vi "Temperature User Interface.vi"() -> ()   [LabVIEW 2023, in "GUI.lvlib" / "Diagnostic.lvlib"]
uses:
  Diagnostic.lvlib
  HardwareAbstractionLayer_LVOOP/Modbus/Modbus_class/Modbus.lvclass
  HardwareAbstractionLayer_LVOOP/Database/SQL Public VI/Control/DB Options.ctl
  HardwareAbstractionLayer_LVOOP/Main/Class Ref.ctl
  HardwareAbstractionLayer_LVOOP/DMM/DMM.lvclass
  HardwareAbstractionLayer_LVOOP/Function Generator/Function Generator.lvclass
  HardwareAbstractionLayer_LVOOP/Oscilloscope/Oscilloscope.lvclass
  HardwareAbstractionLayer_LVOOP/PowerSupply/PowerSupply.lvclass
  HardwareAbstractionLayer_LVOOP/Teststand/Teststand.lvclass
  HardwareAbstractionLayer_LVOOP/Analog Output/AO/AO.lvclass
  HardwareAbstractionLayer_LVOOP/Analog Input/AI/AI.lvclass
  HardwareAbstractionLayer_LVOOP/Database/Database.lvclass
  HardwareAbstractionLayer_LVOOP/Digital Output/DO_class/DO.lvclass
  HardwareAbstractionLayer_LVOOP/Digital Input/DI_class/DI.lvclass
  HardwareAbstractionLayer_LVOOP/PWM Output/PWM Output_class/PWM Output.lvclass
  HardwareAbstractionLayer_LVOOP/PWM Input/PWM Input_class/PWM Input.lvclass
  HardwareAbstractionLayer_LVOOP/NI Switch/NISwitch_class/NISwitch.lvclass
  HardwareAbstractionLayer_LVOOP/CAN/CAN Lib/CAN_class/CAN.lvclass
  HardwareAbstractionLayer_LVOOP/Main/Main.lvclass
panel:
  out "Holding Registers Value":u16[](array[numeric])
  in  "Slave unit ID":u8=1
  out "error out":errorcluster
  in  "Modbus RTU":T1={"unit ID"=1, "serial type"=enum."RTU", "baud rate"=9600, "parity (even)"=2, "flow control (none)"=0, "VISA resource name"=""} {"flow control (none)" items=["None", "XON/XOFF", "RTS/CTS", "XON/XOFF & RTS/CTS", "DTR/DSR", "XON/XOFF & DTR/DSR"]; "parity (even)" items=["None", "Odd", "Even", "Mark", "Space"]}
  in  "error in":errorcluster
  in  "Write Starting Address":u16=8451
  in  "Number of Holding Registers":u16=5
  in  "Read Starting Address":u16=8192
  out "Set Limit Temperature":dbl
  out "Current Temperature":dbl
  in  "Operation":u16(ring) items=["Read", "Write"]
  in  "Set Limit Temperature":i16=27
  in  "Stop":bool caption="Blank"
  in  "Apply":bool caption="Blank"
  # "Temperature Control"
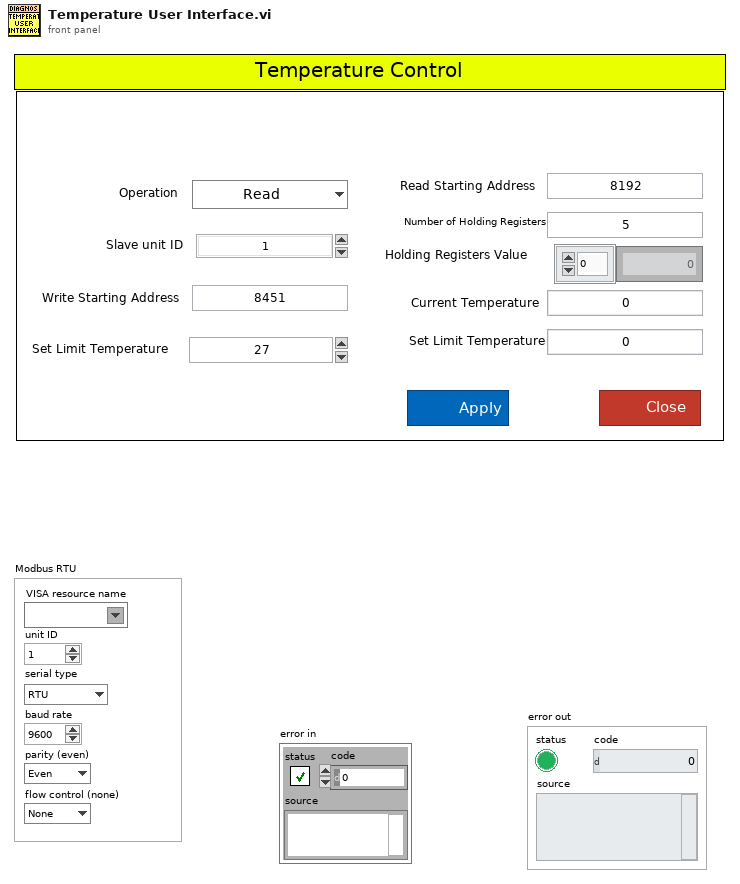
[diagram p1: front panel]
types:
  T1 = cluster{"unit ID":u8, "serial type":enum16{"RTU", "ASCII"}, "baud rate":u32, "parity (even)":u16, "flow control (none)":u16, "VISA resource name":refnum<visa-resource-name>}
  T2 = typedef "HardwareAbstractionLayer_LVOOP.lvlib/Database.lvclass/DB Options.ctl" = enum16{"Init", "Select Data", "Insert Data", "Update Data", "Delete Data", "Execute Query", "Create Schema", "Create Table", "List Tables", "List Columns", "Close"}
  T3 = typedef "HardwareAbstractionLayer_LVOOP.lvlib/Main.lvclass/Class Ref.ctl" = cluster{"DMM":refnum<class "DMM.lvclass">, "Function Generator":refnum<class "Function Generator.lvclass">, "Oscilloscope":refnum<class "Oscilloscope.lvclass">, "PowerSupply":refnum<class "PowerSupply.lvclass">, "Teststand":refnum<class "Teststand.lvclass">, "AO":refnum<class "AO.lvclass">, "AI":refnum<class "AI.lvclass">, "Database":refnum<class "Database.lvclass">, "AO Waveform Generation":refnum<class "AO.lvclass">, "DO":refnum<class "DO.lvclass">, "DI":refnum<class "DI.lvclass">, "PWM Output":refnum<class "PWM Output.lvclass">, "PWM Input":refnum<class "PWM Input.lvclass">, "RelayOutput":refnum<class "NISwitch.lvclass">, "Modbus":refnum<class "Modbus.lvclass">, "CAN":refnum<class "CAN.lvclass">}
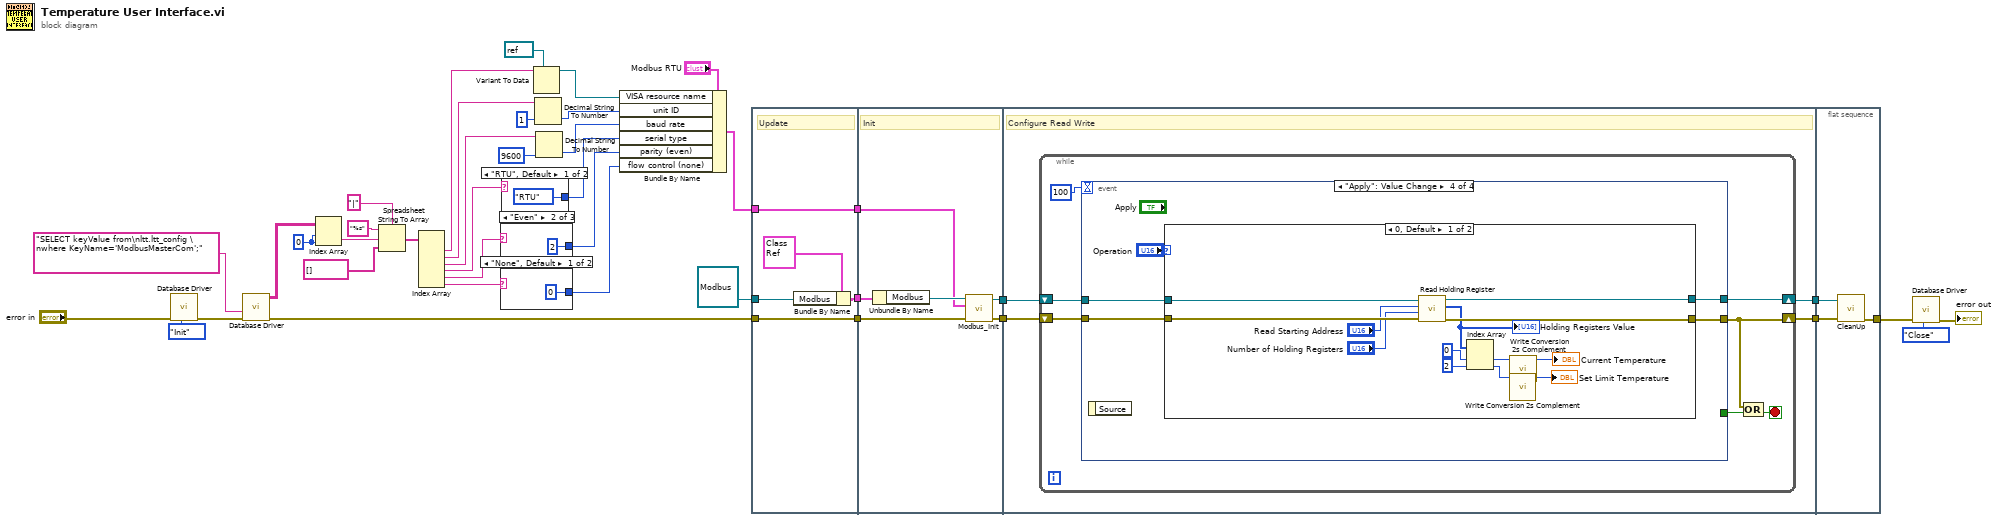
[diagram p0: block diagram]
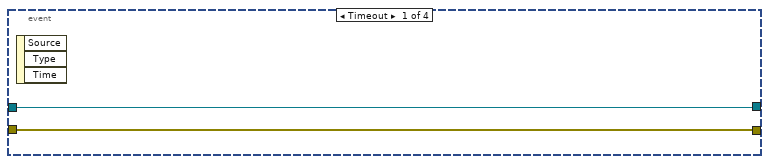
[diagram p2: hidden frame]
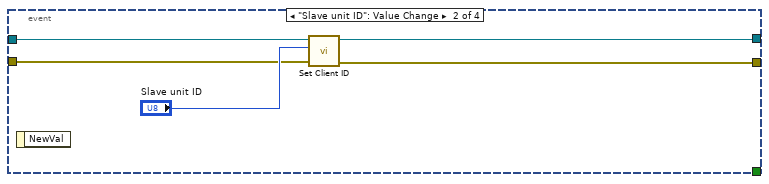
[diagram p3: hidden frame]
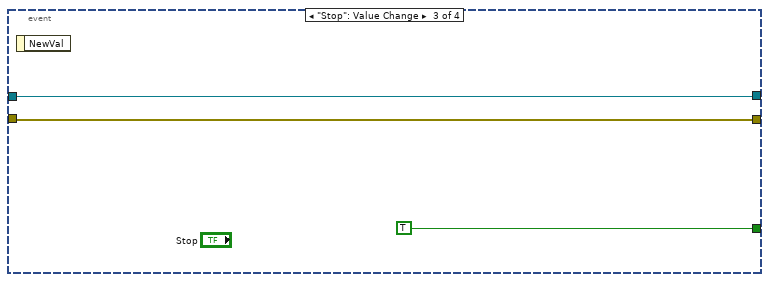
[diagram p4: hidden frame]
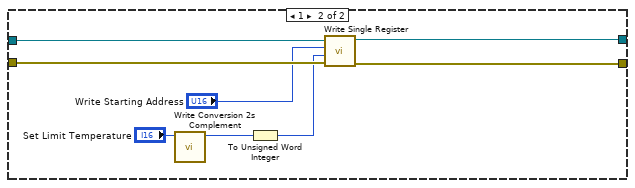
[diagram p5: hidden frame]
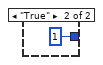
[diagram p6: hidden frame]
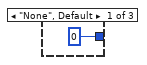
[diagram p7: hidden frame]
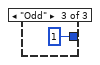
[diagram p8: hidden frame]
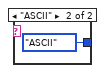
[diagram p9: hidden frame]
diagram:
  w34 = 0 ("index (row)")
  n1 = call "Database Driver.vi"("Options"=DB_Options."Init", "error in"="error in") -> ("error out"=w37:errorcluster)  [unwired: 6 in, 3 out]
  n2 = call "Database Driver.vi"("error in"=w37, "SQL query"="SELECT keyValue from\nltt.ltt_config \nwhere KeyName='ModbusMasterCom';") -> ("error out"=w8:errorcluster, "data"=w35:string[][])  [unwired: 6 in, 2 out]
  n3 = Index Array(array=w35, index (row)=w34, index (col)=w34) -> (element=w33:string)
  n4 = Spreadsheet String To Array(delimiter (Tab)="|" ("format string"), format string="%s", spreadsheet string=w33, array type (2D Dbl)=string[] []) -> (array=w31:string[])
  n5 = Index Array(array=w31) -> (element #1=w16:string, element #2=w29:string, element #3=w26:string, element #4=w23:string, element #5=w21:string, element #6=w20:string)  [unwired: 6 in]
  n6 = case shown="\"Even\"" w21 {
    tunnel: [u16 0 ("parity (even)") u16 2 ("parity (even)") u16 1 ("parity (even)")] -> w19
    frame "None", Default {
    }
    frame "Even" {
    }
    frame "Odd" {
    }
  }
  n7 = case shown="\"None\", Default" w20 {
    tunnel: [u16 0 ("flow control (none)") u16 1 ("flow control (none)")] -> w18
    frame "None", Default {
    }
    frame "True" {
    }
  }
  n8 = case shown="\"RTU\", Default" w23 {
    tunnel: [enum16{"RTU", "ASCII"}."RTU" ("serial type") enum16{"RTU", "ASCII"}."ASCII" ("serial type")] -> w22
    frame "RTU", Default {
    }
    frame "ASCII" {
    }
  }
  n9 = Variant To Data(type=refnum<visa-resource-name> refnum ("VISA resource name"), Variant=w16) -> (data=w15:refnum<visa-resource-name>)  [unwired: 1 in, 1 out]
  n10 = Decimal String To Number(string=w29, default (0L)=u8 1 ("unit ID")) -> (number=w27:u8)  [unwired: 1 in, 1 out]
  n11 = Decimal String To Number(string=w26, default (0L)=u32 9600 ("baud rate")) -> (number=w25:u32)  [unwired: 1 in, 1 out]
  n12 = Bundle By Name(cluster="Modbus RTU", "VISA resource name"=w15, "unit ID"=w27, "baud rate"=w25, "serial type"=w22, "parity (even)"=w19, "flow control (none)"=w18) -> (w10:T1)
  n13 = flat-sequence {
    tunnel: refnum<class "Modbus.lvclass"> refnum ("HardwareAbstractionLayer_LVOOP.lvlib:Modbus") -> [w51]
    tunnel: [w50] -> w12
    tunnel: w10 -> [w49]
    tunnel: [w49] -> w9
    tunnel: w8 -> [w48]
    tunnel: [w48] -> w7
    tunnel: w12 -> [w58]
    tunnel: [w56] -> w11
    tunnel: w9 -> [w55]
    tunnel: w7 -> [w54]
    tunnel: [w53] -> w6
    tunnel: w11 -> [w62]
    tunnel: w6 -> [w61]
    tunnel: [w60] -> w5
    tunnel: [w59] -> w4
    tunnel: w5 -> [w108]
    tunnel: w4 -> [w107]
    tunnel: [w106] -> w3
    frame #0 {
      # "Update"
      n14 = Bundle By Name(cluster=T3 {"DMM"=refnum, "Function Generator"=refnum, "Oscilloscope"=refnum, "PowerSupply"=refnum, "Teststand"=refnum, "AO"=refnum, "AI"=refnum, "Database"=refnum, "AO Waveform Generation"=refnum, "DO"=refnum, "DI"=refnum, "PWM Output"=refnum, "PWM Input"=refnum, "RelayOutput"=refnum, "Modbus"=refnum, "CAN"=refnum} ("Class Cluster"), "Modbus"=w51) -> (w50:T3)
    }
    frame #1 {
      # "Init"
      n15 = Unbundle By Name(w58) -> ("Modbus"=w57:refnum<class "Modbus.lvclass">)
      n16 = call "Modbus_Init.vi"("error in (no error)"=w54, "Modbus RTU"=w55, "object in"=w57) -> ("error out"=w53:errorcluster, "object out"=w56:refnum<class "Modbus.lvclass">)  [unwired: 7 in]
    }
    frame #2 {
      # "Configure Read Write"
      n17 = while {
        shift-right: [w65] -> w60
        shift-left: w62 -> [w67]
        shift-right: [w63] -> w59
        shift-left: w61 -> [w66]
        stop <- w64 stop-if-true
        n18 = event shown="[3] \"Apply\": Value Change" {
          selector: _ -> [_ _ _ _]
          dyn-events: _ -> [_ _ _ _]
          timeout: 100 -> [_ _ _ _]
          tunnel: [_ _ TRUE _] -> w68
          tunnel: w67 -> [w71 w75 w78 w83]
          tunnel: w66 -> [w70 w72 w77 w82]
          tunnel: [w71 w74 w78 w81] -> w65
          tunnel: [w70 w73 w77 w80] -> w63
          event Timeout {
            n19 = event-data() -> ()  [unwired: 1 in, 3 out]
          }
          event "Slave unit ID": Value Change {
            n20 = event-data() -> ()  [unwired: 1 in, 1 out]
            n21 = call-dynamic "Set Client ID.vi"("error in (no error)"=w72, "Slave unit ID"="Slave unit ID", "Modbus in"=w75) -> ("error out"=w73:errorcluster, "Modbus out"=w74:refnum<class "Modbus.lvclass">)  [unwired: 7 in]
          }
          event "Stop": Value Change {
            n22 = event-data() -> ()  [unwired: 1 in, 1 out]
          }
          event "Apply": Value Change {
            n23 = event-data() -> ()  [unwired: 1 in, 1 out]
            n24 = case shown="0, Default" "Operation" {
              tunnel: w83 -> [w97 w105]
              tunnel: w82 -> [w96 w104]
              tunnel: [w95 w103] -> w81
              tunnel: [w94 w102] -> w80
              frame 0, Default {
                n25 = call-dynamic "Read Holding Register.vi"("error in (no error)"=w96, "number of inputs"="Number of Holding Registers", "starting address"="Read Starting Address", "Modbus in"=w97) -> ("error out"=w94:errorcluster, "register values"=w89:u16[], "Modbus out"=w95:refnum<class "Modbus.lvclass">)  [unwired: 5 in]
                "Holding Registers Value" <- w89
                n26 = Index Array(array=w89, index #1=0 ("index"), index #2=2 ("index")) -> (element #1=w86:u16, element #2=w88:u16)
                n27 = call "Write Conversion 2s Complement.vi"("Set Data Input"=w88) -> ("Coversion Data Output"=→"Set Limit Temperature":i16)  [unwired: 10 in]
                n28 = call "Write Conversion 2s Complement.vi"("Set Data Input"=w86) -> ("Coversion Data Output"=→"Current Temperature":i16)  [unwired: 10 in]
              }
              frame 1 {
                n29 = call "Write Conversion 2s Complement.vi"("Set Data Input"="Set Limit Temperature") -> ("Coversion Data Output"=w99:i16)  [unwired: 10 in]
                n30 = To Unsigned Word Integer(number=w99) -> (unsigned 16bit integer=w98:u16)
                n31 = call-dynamic "Write Single Register.vi"("error in (no error)"=w104, "Write Value"=w98, "Write address"="Write Starting Address", "Modbus in"=w105) -> ("error out"=w102:errorcluster, "Modbus out"=w103:refnum<class "Modbus.lvclass">)  [unwired: 6 in]
              }
            }
          }
        }
        n32 = Compound Arithmetic op=OR(w63, w68) -> (w64:bool)
      }
    }
    frame #3 {
      n33 = call-dynamic "CleanUp.vi"("object in"=w108, "error in (no error)"=w107) -> ("error out"=w106:errorcluster)  [unwired: 16 in, 1 out]
    }
  }
  n34 = call "Database Driver.vi"("Options"=DB_Options."Close", "error in"=w3) -> ("error out"=→"error out":errorcluster)  [unwired: 6 in, 3 out]
